vi "resistanceToConductivity.vi"(11 "ELECTRIC RESISTANCE":dbl) -> (3 "Numeric":dbl)   [LabVIEW 2020]
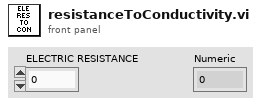
[diagram p1: front panel]
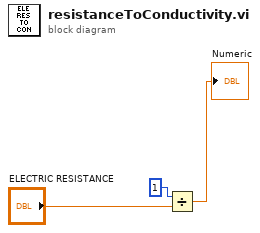
[diagram p0: block diagram]
diagram:
  n1 = Divide(x=1, y="ELECTRIC RESISTANCE") -> (x/y=→"Numeric":dbl)
